vi "Generate OD data.vi"(4 "dark":u16[][](array[numeric]), 5 "light":u16[][](array[numeric]), 6 "atom":u16[][](array[numeric])) -> (2 "OD image":u16[][](array[numeric]))   [LabVIEW 2015]
panel:
  out "x*y":dbl[][](array[numeric])
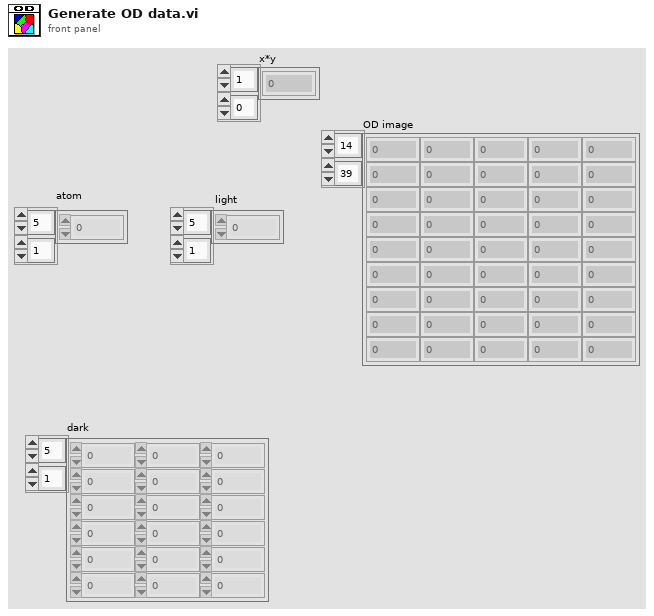
[diagram p1: front panel]
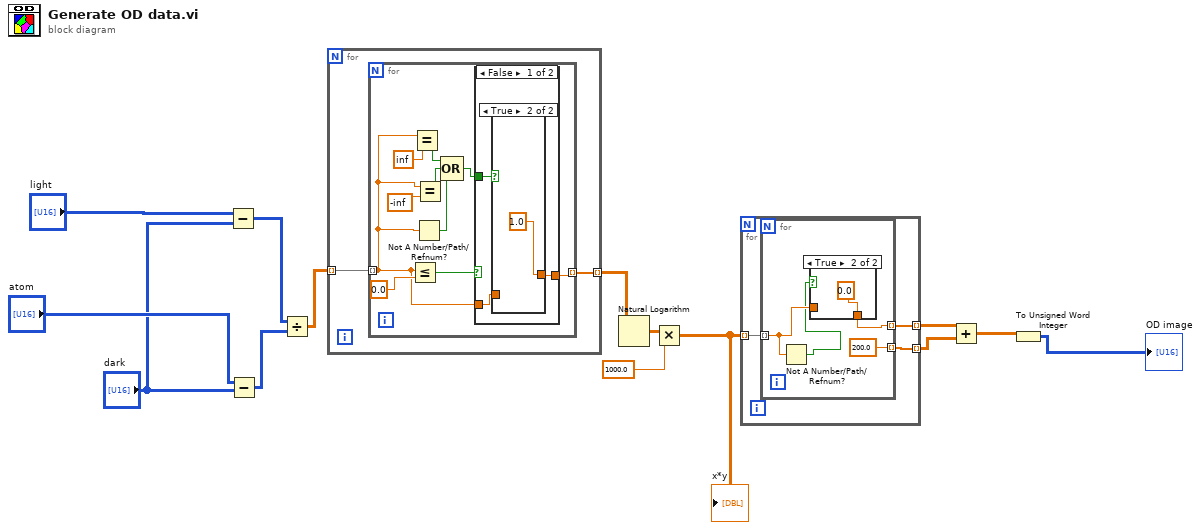
[diagram p0: block diagram]
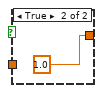
[diagram p4: hidden frame]
diagram:
  n1 = Subtract(x="light", y="dark") -> (x-y=w11:u16[][])
  n2 = Subtract(x="atom", y="dark") -> (x-y=w10:u16[][])
  n3 = Divide(x=w11, y=w10) -> (x/y=w9:dbl[][])
  n4 = for {
    tunnel: w9 -> [w16] mode=indexing
    tunnel: [w15] -> w8 mode=indexing
    n5 = for {
      tunnel: w16 -> [w18] mode=indexing
      tunnel: [w24] -> w15 mode=indexing
      n6 = Less Or Equal?(x=w18, y=0.0) -> (x <= y?=w25:bool)
      n7 = Equal?(x=w18, y=inf) -> (x = y?=w21:bool)
      n8 = Not A Number/Path/Refnum?(number/path/refnum=w18) -> (NaN/Path/Refnum?=w17:bool)
      n9 = Equal?(x=w18, y=-inf) -> (x = y?=w20:bool)
      n10 = Compound Arithmetic op=OR(w21, w20, w17) -> (w19:bool)
      n11 = case shown="False" w25 {
        tunnel: w18 -> [w27 _]
        tunnel: [w28 1.0 ("数值")] -> w24
        tunnel: w19 -> [w29 _]
        frame False {
          n12 = case shown="True" w29 {
            tunnel: [w30 1.0 ("y")] -> w28
            tunnel: w27 -> [w30 _]
            frame False {
            }
            frame True {
            }
          }
        }
        frame True {
        }
      }
    }
  }
  n13 = Natural Logarithm(1:w8) -> (0:w6:dbl[][])
  n14 = Multiply(x=w6, y=1000.0) -> (x*y=w5:dbl[][])
  "x*y" <- w5
  n15 = for {
    tunnel: [w35] -> w4 mode=indexing
    tunnel: w5 -> [w34] mode=indexing
    tunnel: [w33] -> w3 mode=indexing
    n16 = for {
      tunnel: [w39] -> w35 mode=indexing
      tunnel: w34 -> [w38] mode=indexing
      tunnel: [200.0 ("y")] -> w33 mode=indexing
      n17 = Not A Number/Path/Refnum?(number/path/refnum=w38) -> (NaN/Path/Refnum?=w37:bool)
      n18 = case shown="True" w37 {
        tunnel: [w40 0.0 ("y")] -> w39
        tunnel: w38 -> [w40 _]
        frame False {
        }
        frame True {
        }
      }
    }
  }
  n19 = Add(x=w4, y=w3) -> (x+y=w2:dbl[][])
  n20 = To Unsigned Word Integer(number=w2) -> (unsigned 16bit integer=→"OD image":u16[][])
